vi "Audio Config.vi"(11 "Shutdown Event":refnum<user-event>) -> ()   [LabVIEW 2019, in "User Interface.lvlib"]
doc: "Audio config sub panel. The audio output configuration is set here and updated in the Audio Output loop when Apply is clicked.\n\n<b>Execution System:</b> User Interface"
uses:
  User Interface.lvlib
  Custom Graphics/Ring.Black.ctl
  Custom Graphics/Button.Large.ctl
  Audio Output/Audio Output Config.ctl
  Audio Output/Audio Output Info.ctl
  Packed Libraries/Messaging.lvlibp/Message Cluster.ctl
  Audio Output/Audio Output.lvlib
  Packed Libraries/Messaging.lvlibp
panel:
  out "Version":string
  in  "Apply":T1
  in  "Headphone Output":T2=65535 items=["(Disabled)"=65535, "Speakers (High Definition Audio Device)"=0]
  in  "Master Output":T2=65535 items=["(Disabled)"=65535, "Speakers (High Definition Audio Device)"=0]
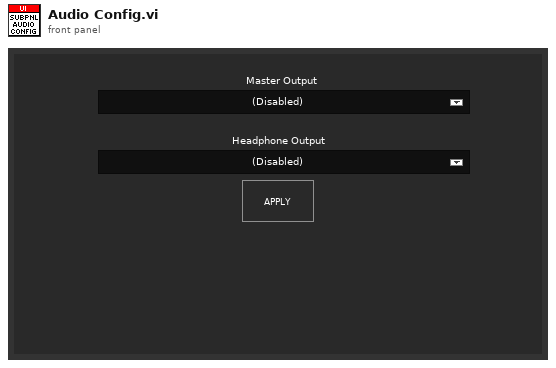
[diagram p1: front panel]
types:
  T1 = typedef "User Interface.lvlib/Button.Large.ctl" = bool
  T2 = typedef "User Interface.lvlib/Ring.Black.ctl" = u16
  T3 = typedef "Audio Output.lvlib/Audio Output Config.ctl" = cluster{"Master":T4, "Headphones":T4}
  T4 = typedef "Audio Output.lvlib/Audio Output Info.ctl" = cluster{"Enable":bool, "Output ID":i32}
  T5 = typedef "Messaging.lvlibp/Message Cluster.ctl" = cluster{"Event":string, "Source":string, "Target":string, "Data":variant}
  T6 = typedef "LVStringsAndValuesArrayTypeDef_U16.ctl" = cluster{"String":string, "Value":u16}[]
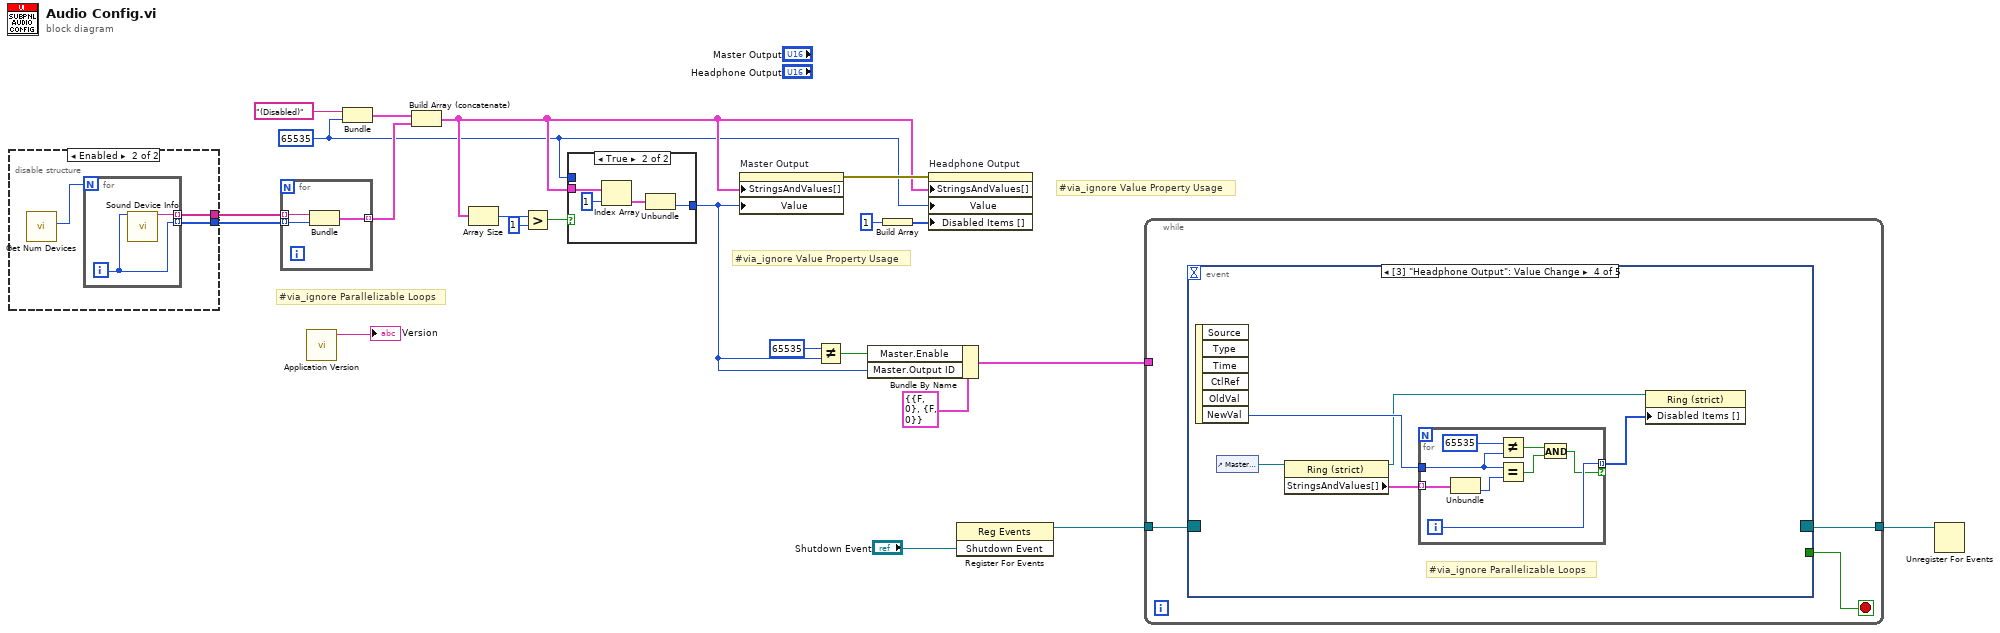
[diagram p0: block diagram]
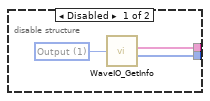
[diagram p2: hidden frame]
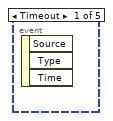
[diagram p3: hidden frame]
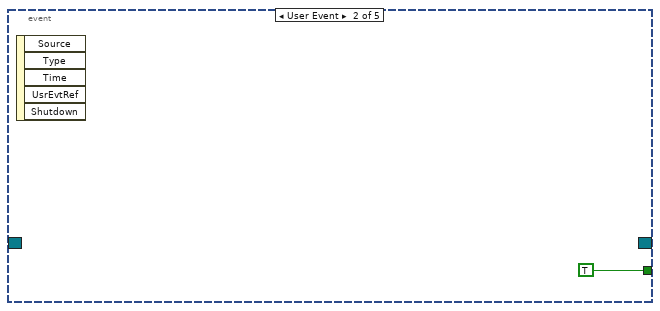
[diagram p4: hidden frame]
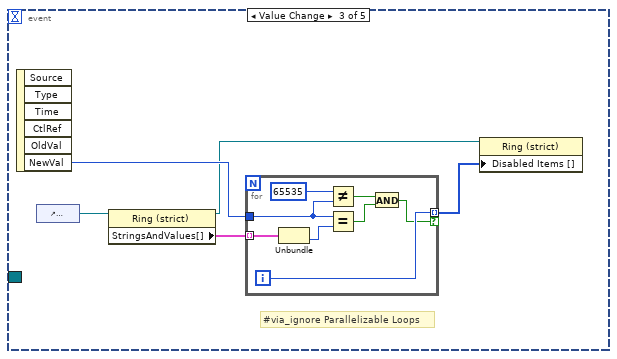
[diagram p5: hidden frame]
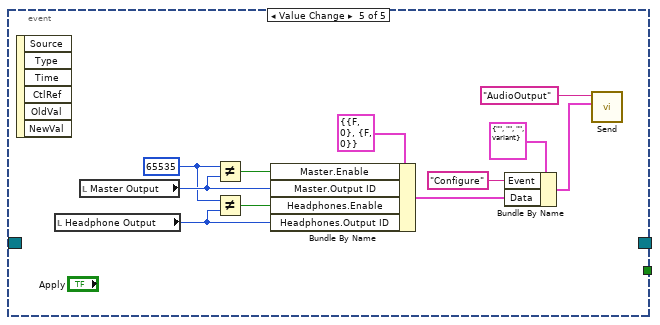
[diagram p6: hidden frame]
diagram:
  w12 = u16 65535
  # "#via_ignore Value Property Usage"
  # "#via_ignore Value Property Usage"
  # "#via_ignore Parallelizable Loops"
  n1 = disable-structure shown="Enabled" {
    disable-tunnel: [w24 w28] -> w21
    disable-tunnel: [w23 w27] -> w20
    frame Disabled {
      w25 = u16 1 items=["Input", "Output", "Loopback", "ASIO input", "ASIO output", "Record (WASAPI)", "Play (WASAPI)"] ("Direction (Input)")
      n2 = call "WaveIO_GetInfo.vi"("Direction (Input)"=w25) -> ("Dev Names"=w24:string[], "IDDev"=w23:i32[])  [unwired: 2 out]
    }
    frame Enabled {
      n3 = call <vilib>:"Get Num Devices.vi"() -> ("Number of Output Devices"=w26:i32)  [unwired: 9 in, 2 out]
      n4 = for {
        N: w26 -> [_]
        tunnel: [w30] -> w28 mode=indexing
        tunnel: [w29] -> w27 mode=indexing
        i -> [w29]
        n5 = call <vilib>:"Sound Device Info.vi"("device"=w29) -> ("Device Name"=w30:string)  [unwired: 12 in, 2 out]
      }
    }
  }
  n6 = for {
    tunnel: w21 -> [w33] mode=indexing
    tunnel: w20 -> [w32] mode=indexing
    tunnel: [w31] -> w17 mode=indexing
    n7 = Bundle("Device Name"=w33, w32) -> (w31:cluster{"Device Name":string, i32})  [unwired: 1 in]
  }
  n8 = call "Application Version.vi"() -> ("Application Version"=→"Version":string)  [unwired: 11 in]
  n9 = Bundle("(Disabled)", w12) -> (w18:cluster{string, u16})  [unwired: 1 in]
  n10 = Build Array (concatenate)(w18, w17) -> (w13:cluster{"Device Name":string, i32}[])
  n11 = Array Size(array=w13) -> (size(s)=w16:i32)
  n12 = Greater?(x=w16, y=1) -> (0:w14:bool)
  n13 = case shown="True" w14 {
    tunnel: w13 -> [_ w38]
    tunnel: [w34 w35] -> w6
    tunnel: w12 -> [w34 _]
    frame False {
    }
    frame True {
      n14 = Index Array(array=w38, index=1) -> (element=w36:cluster{"Device Name":string, i32})
      n15 = Unbundle(w36) -> (w35:i32)  [unwired: 1 out]
    }
  }
  n16 = property on="Master Output" class="Ring (strict)"("StringsAndValues[]"=w13, "Value"=w6) -> (error out=w22:errorcluster)  [unwired: 2 in, 1 out]
  n17 = Not Equal?(x=65535, y=w6) -> (x != y?=w7:bool)
  n18 = Bundle By Name(cluster=T3 {"Master"={"Enable"=FALSE, "Output ID"=0}, "Headphones"={"Enable"=FALSE, "Output ID"=0}} ("Audio Output Config"), "Master.Enable"=w7, "Master.Output ID"=w6) -> (w5:T3)
  n19 = Build Array(1 ("y")) -> (w11:i32[])
  n20 = property on="Headphone Output" class="Ring (strict)"(error in=w22, "StringsAndValues[]"=w13, "Value"=w12, "Disabled Items []"=w11) -> ()  [unwired: 1 in, 2 out]
  n21 = register-events("Shutdown Event") -> (reference out=w3:refnum<event-registration>)  [unwired: 2 in, 1 out]
  n22 = while {
    tunnel: w5 -> [_]
    tunnel: w3 -> [w41]
    tunnel: [w40] -> w2
    stop <- w39 stop-if-true
    n23 = event shown="[3] \"Headphone Output\": Value Change" {
      selector: w41 -> [_ _ _ _ _]
      dyn-events: [_ _ _ _ _] -> w40
      timeout: _ -> [_ _ _ _ _]
      tunnel: [_ TRUE _ _ _] -> w39
      event Timeout {
        n24 = event-data() -> ()  [unwired: 1 in, 3 out]
      }
      event User Event {
        n25 = event-data() -> ()  [unwired: 1 in, 5 out]
      }
      event Value Change {
        # "#via_ignore Parallelizable Loops"
        n26 = event-data() -> ("NewVal"=w45:T2)  [unwired: 1 in, 5 out]
        n27 = control-ref of="Headphone Output"() -> (w47:refnum<vi>)
        n28 = property class="Ring (strict)"(reference=w47) -> (reference out=w43:refnum<vi>, "StringsAndValues[]"=w46:T6)  [unwired: 1 in, 1 out]
        n29 = for {
          tunnel: w46 -> [w55] mode=indexing
          tunnel: w45 -> [w51]
          tunnel: [w53] -> w44 mode=indexing if=w48
          i -> [w53]
          n30 = Unbundle(w55) -> ("Value"=w54:u16)  [unwired: 1 out]
          n31 = Not Equal?(x=65535, y=w51) -> (x != y?=w49:bool)
          n32 = Equal?(x=w51, y=w54) -> (x = y?=w52:bool)
          n33 = And(x=w49, y=w52) -> (x .and. y?=w48:bool)
        }
        n34 = property class="Ring (strict)"(reference=w43, "Disabled Items []"=w44) -> ()  [unwired: 1 in, 2 out]
      }
      event Value Change {
        # "#via_ignore Parallelizable Loops"
        n35 = event-data() -> ("NewVal"=w59:T2)  [unwired: 1 in, 5 out]
        n36 = control-ref of="Master Output"() -> (w56:refnum<vi>)
        n37 = property class="Ring (strict)"(reference=w56) -> (reference out=w57:refnum<vi>, "StringsAndValues[]"=w60:T6)  [unwired: 1 in, 1 out]
        n38 = for {
          tunnel: w60 -> [w68] mode=indexing
          tunnel: w59 -> [w64]
          tunnel: [w66] -> w58 mode=indexing if=w61
          i -> [w66]
          n39 = Unbundle(w68) -> ("Value"=w67:u16)  [unwired: 1 out]
          n40 = Not Equal?(x=65535, y=w64) -> (x != y?=w62:bool)
          n41 = Equal?(x=w64, y=w67) -> (x = y?=w65:bool)
          n42 = And(x=w62, y=w65) -> (x .and. y?=w61:bool)
        }
        n43 = property class="Ring (strict)"(reference=w57, "Disabled Items []"=w58) -> ()  [unwired: 1 in, 2 out]
      }
      event Value Change {
        w69 = u16 65535
        n44 = event-data() -> ()  [unwired: 1 in, 6 out]
        n45 = local read "Headphone Output"() -> (w70:T2)
        n46 = local read "Master Output"() -> (w72:T2)
        n47 = Not Equal?(x=w69, y=w72) -> (x != y?=w73:bool)
        n48 = Not Equal?(x=w69, y=w70) -> (x != y?=w71:bool)
        n49 = Bundle By Name(cluster=T3 {"Master"={"Enable"=FALSE, "Output ID"=0}, "Headphones"={"Enable"=FALSE, "Output ID"=0}} ("Audio Output Config"), "Master.Enable"=w73, "Master.Output ID"=w72, "Headphones.Enable"=w71, "Headphones.Output ID"=w70) -> (w74:T3)
        n50 = Bundle By Name(cluster=T5 {"Event"="", "Source"="", "Target"="", "Data"=variant} ("Message"), "Event"="Configure" ("Type"), "Data"=w74) -> (w77:T5)
        n51 = call "Send.vi"("Message"=w77, "Queue Name"="AudioOutput") -> ()  [unwired: 9 in, 1 out]
      }
    }
  }
  n52 = Unregister For Events(event registration refnum=w2) -> ()  [unwired: 1 in, 1 out]
